vi "TagContainer-Free.vi"(8 "error in (no error)":errorcluster, 11 "TagContainer":T1) -> (0 "error out":errorcluster)   [LabVIEW 2017, in "TagContainer.lvlib"]
uses:
  TagContainer.lvlib
  Typedef/TagContainer.ctl
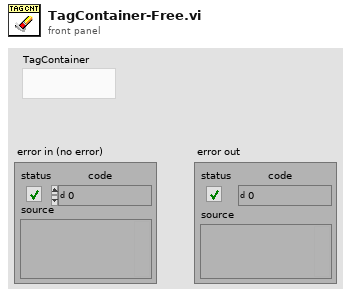
[diagram p1: front panel]
types:
  T1 = typedef "TagContainer.lvlib/TagContainer.ctl" = refnum<k1>
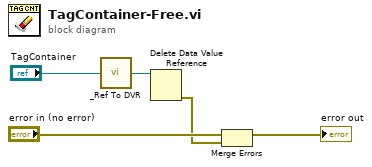
[diagram p0: block diagram]
diagram:
  n1 = call "_Ref To DVR.vi"("TagContainer"="TagContainer") -> ("DVR"=w2:refnum<data-value>)
  n2 = Delete Data Value Reference(data value reference=w2) -> (error out=w3:errorcluster)  [unwired: 1 in, 1 out]
  n3 = Merge Errors("error in (no error)", w3) -> (→"error out":errorcluster)
